vi "Latch if True.vi"(8 "Switch State":bool, 11 "Current State":bool) -> (2 "State Out":bool)   [LabVIEW 2021]
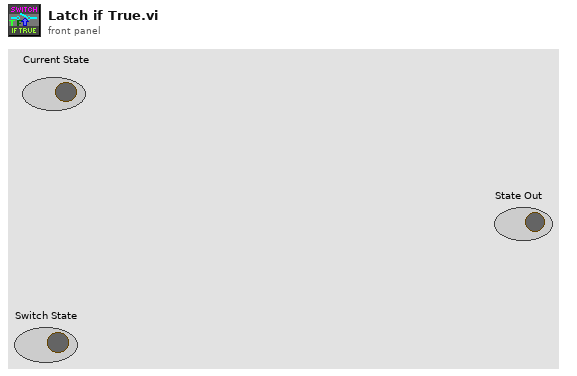
[diagram p1: front panel]
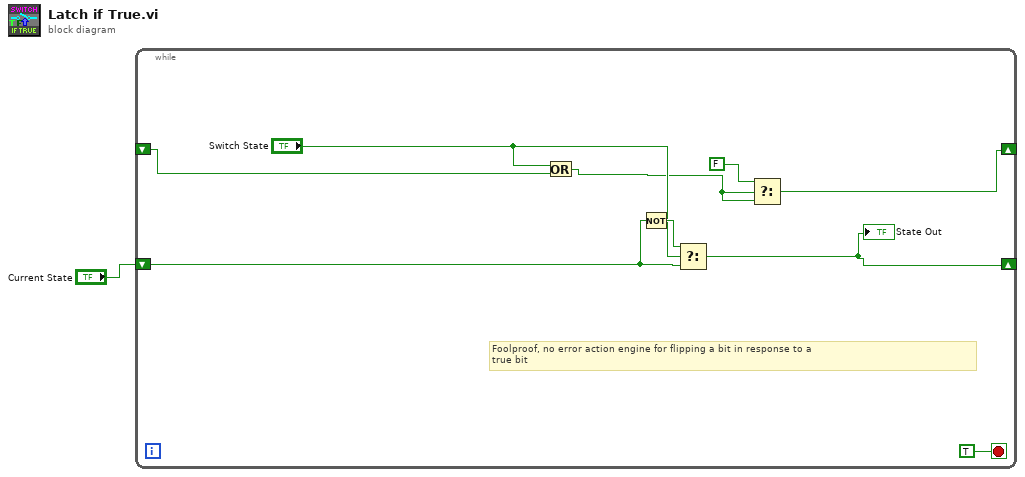
[diagram p0: block diagram]
diagram:
  n1 = while {
    shift-right: [w8] -> _
    shift-left: "Current State" -> [w9]
    shift-right: [w6] -> _
    shift-left: _ -> [w4]
    stop <- TRUE stop-if-true
    # "Foolproof, no error action engine for flipping a bit in response to a\ntrue bit"
    n2 = Or(x="Switch State", y=w4) -> (x .or. y?=w3:bool)
    n3 = Not(x=w9) -> (.not. x?=w10:bool)
    n4 = Select(t=w10, s="Switch State", f=w9) -> (s? t:f=w8:bool)
    "State Out" <- w8
    n5 = Select(t=FALSE, s=w3, f=w3) -> (s? t:f=w6:bool)
  }
